vi "RUSHKinectCalibrate.vi"(8 "Arm Drive Min in (Reverse)":dbl, 9 "Arm Drive Max in (Forward)":dbl, 10 "Z Wrist Left":dbl, 11 "Z Wrist Right":dbl) -> (0 "Z Wrist Left":sgl, 1 "Z Wrist Right":sgl, 2 "Calibrating":bool, 3 "Result":T1(ring), 4 "Arm Drive Min out (Reverse)":dbl, 5 "Arm Drive Max out (Forward)":dbl)   [LabVIEW 2011]
uses:
  <vilib>/addons/Kinect/Skeleton Vertex Index.ctl
panel:
  out "Go to Calibrate":bool
  in  "Muscle Tolerance":dbl=0.05
  out "In The Middle ?":bool
  out "?":dbl(slide) scale=2.4213576316833496..2.7618839740753174
  out "Current Max":dbl
  out "Current Min":dbl
  out "Average Current Position (Both Hands)":dbl
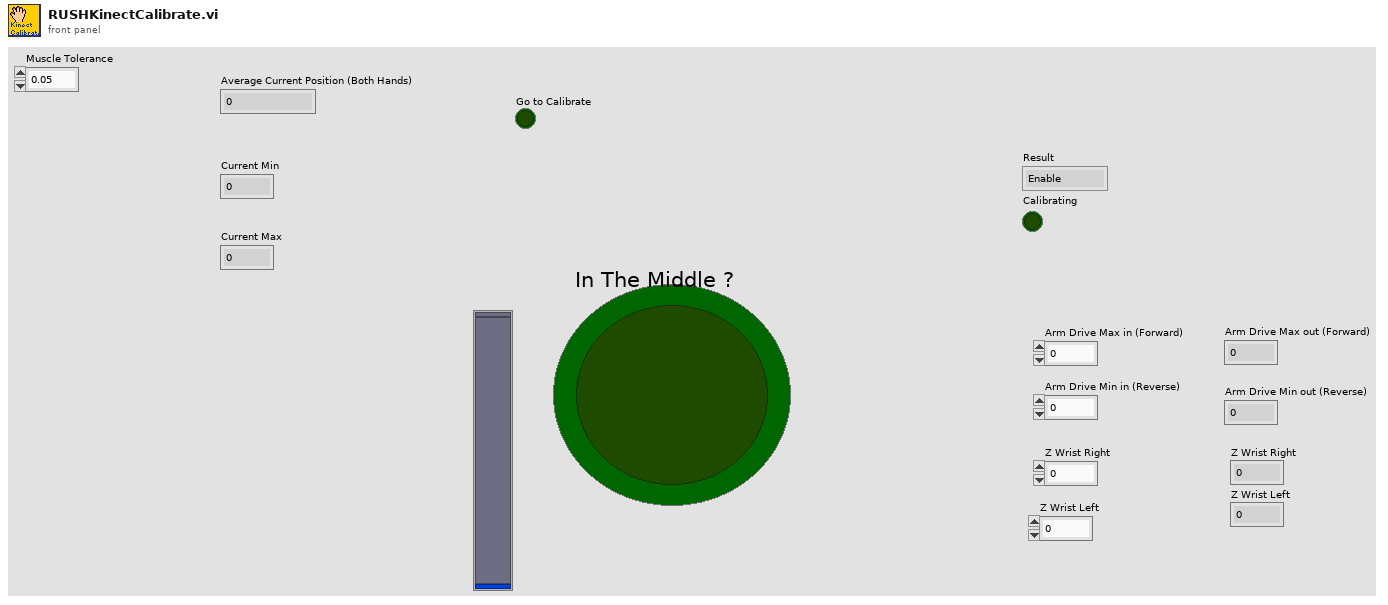
[diagram p1: front panel]
types:
  T1 = enum16{"Enable", "Set/Reset", "Run Timer", "Read/Store"}
  T2 = typedef "Skeleton Vertex Index.ctl" = i32
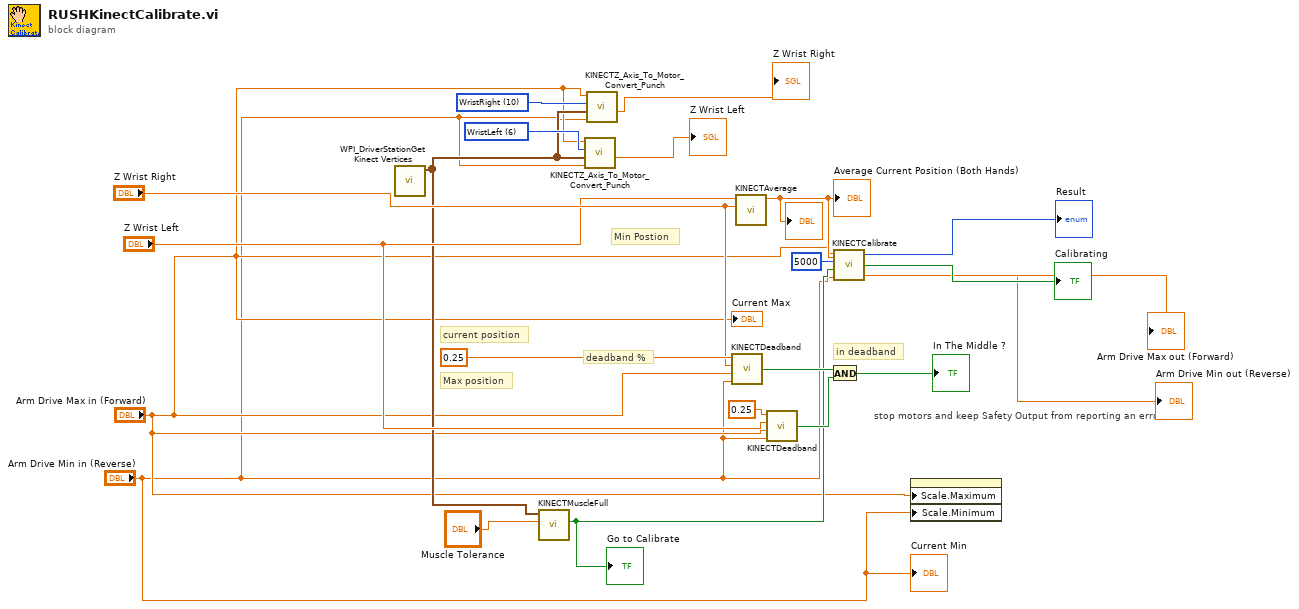
[diagram p0: block diagram]
diagram:
  w21 = T2 10 items=["HipCenter", "Spine", "ShoulderCenter", "Head", "ShoulderLeft", "ElbowLeft", "WristLeft", "HandLeft", "ShoulderRight", "ElbowRight", "WristRight", "HandRight", "HipLeft", "KneeLeft", "AnkleLeft", "FootLeft", "HipRight", "KneeRight", "AnkleRight", "FootRight"] ("Skeleton Joints")
  w22 = T2 6 items=["HipCenter", "Spine", "ShoulderCenter", "Head", "ShoulderLeft", "ElbowLeft", "WristLeft", "HandLeft", "ShoulderRight", "ElbowRight", "WristRight", "HandRight", "HipLeft", "KneeLeft", "AnkleLeft", "FootLeft", "HipRight", "KneeRight", "AnkleRight", "FootRight"] ("Skeleton Joints")
  # "deadband %"
  # "Min Postion"
  # "Max position"
  # "current position"
  # "in deadband"
  # "stop motors and keep Safety Output from reporting an error"
  n1 = call <vilib>:"WPI_DriverStationGet Kinect Vertices.vi"() -> ("Skeleton Vertices"=w6:cluster{"x":sgl, "y":sgl, "z":sgl}[])  [unwired: 10 in, 1 out]
  n2 = call "KINECTMuscleFull.vi"("Muscle Tolerance"="Muscle Tolerance", "Skeleton Vertices"=w6) -> ("Go to Calibrate"=w5:bool)  [unwired: 9 in]
  "Go to Calibrate" <- w5
  n3 = call "KINECTZ_Axis_To_Motor_Convert_Punch.vi"("Arm Drive Min (Reverse)"="Arm Drive Min in (Reverse)", "Skeleton Vertices"=w6, "Wrist Input"=w22, "Arm Drive Max (Forward)"="Arm Drive Max in (Forward)") -> ("Z Axis Out"=→"Z Wrist Left":sgl)  [unwired: 5 in, 2 out]
  n4 = call "KINECTZ_Axis_To_Motor_Convert_Punch.vi"("Arm Drive Min (Reverse)"="Arm Drive Min in (Reverse)", "Skeleton Vertices"=w6, "Wrist Input"=w21, "Arm Drive Max (Forward)"="Arm Drive Max in (Forward)") -> ("Z Axis Out"=→"Z Wrist Right":sgl)  [unwired: 5 in, 2 out]
  n5 = call "KINECTDeadband.vi"("Min"="Arm Drive Min in (Reverse)", "Max"="Arm Drive Max in (Forward)", "Current Position"="Z Wrist Right", "Deadband %"=0.25 ("x")) -> ("In Range?"=w19:bool)
  n6 = call "KINECTAverage.vi"("Min"="Z Wrist Right", "Max"="Z Wrist Left") -> ("Average"=w15:dbl)  [unwired: 8 in, 1 out]
  "Average Current Position (Both Hands)" <- w15
  "?" <- w15
  n7 = call "KINECTDeadband.vi"("Min"="Arm Drive Min in (Reverse)", "Max"="Arm Drive Max in (Forward)", "Current Position"="Z Wrist Left", "Deadband %"=0.25 ("x")) -> ("In Range?"=w17:bool)
  n8 = And(x=w19, y=w17) -> (x .and. y?=→"In The Middle ?":bool)
  n9 = call "KINECTCalibrate.vi"("Arm Drive Min in (Reverse)"="Arm Drive Min in (Reverse)", "Enable Calibration"=w5, "Current Value"=w15, "Wait Time (ms)"=u32 5000, "Arm Drive Max in (Forward)"="Arm Drive Max in (Forward)") -> ("Arm Drive Min out (Reverse)"=→"Arm Drive Min out (Reverse)":dbl, "Arm Drive Max out (Forward)"=→"Arm Drive Max out (Forward)":dbl, "Calibrating"=→"Calibrating":bool, "Result"=→"Result":T1)  [unwired: 2 in]
  n10 = property class="Slide (strict)"("Scale.Maximum"="Arm Drive Max in (Forward)", "Scale.Minimum"="Arm Drive Min in (Reverse)") -> ()  [unwired: 2 in, 2 out]
  "Current Min" <- "Arm Drive Min in (Reverse)"
  "Current Max" <- "Arm Drive Max in (Forward)"
